vi "UpdateFile.vi"(8 "error in (no error)":errorcluster, 10 "Account Info":T1, 11 "path":path) -> (0 "error out":errorcluster)   [LabVIEW 2017]
doc: "This VI is responsible for updating the file database with the latest values."
uses:
  <vilib>/Utility/file.llb/Write To Spreadsheet File (string).vi
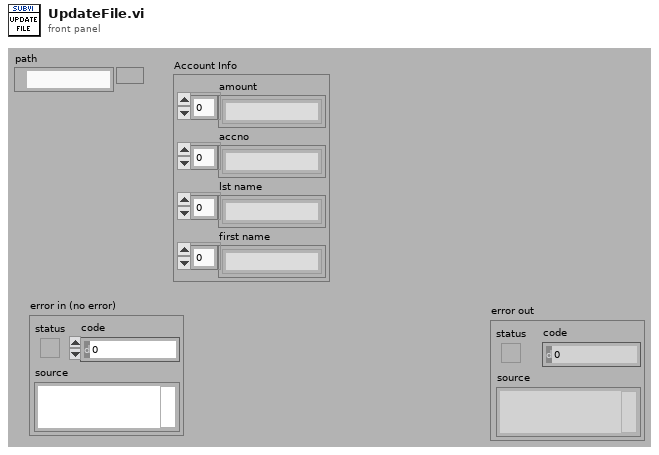
[diagram p1: front panel]
types:
  T1 = cluster{"amount":string[], "accno":string[], "lst name":string[], "first name":string[]}
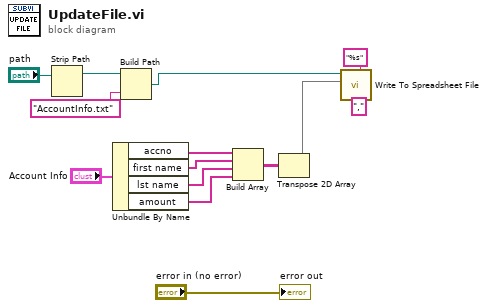
[diagram p0: block diagram]
diagram:
  n1 = Strip Path(path="path") -> (stripped path=w13:path)  [unwired: 1 out]
  n2 = Unbundle By Name("Account Info") -> ("accno"=w10:string[], "first name"=w9:string[], "lst name"=w8:string[], "amount"=w7:string[])
  n3 = Build Path(base path=w13, name or relative path="AccountInfo.txt") -> (appended path=w12:path)
  n4 = Build Array(w10, w9, w8, w7) -> (w4:string[][])
  n5 = Transpose 2D Array(2D array=w4) -> (transposed array=w3:string[][])
  n6 = call-poly <vilib>:"Write To Spreadsheet File.vi"("delimiter (\\t)"="," ("delimiter (\\t)"), "format (%s)"="%s", "2D data"=w3, "file path (dialog if empty)"=w12) -> ()  [unwired: 4 in, 1 out]
  "error out" <- "error in (no error)"
